vi "Move VI to Subpanel.vi"(8 "error in":errorcluster, 9 "VI name":string, 10 "subpanel tag":string, 11 "state in":T1) -> (0 "error out":errorcluster, 3 "state out":T1)   [LabVIEW 2010, in "NI_SE_Config Front Panel Layout.lvlib"]
uses:
  NI_SE_Config Front Panel Layout.lvlib
  State.ctl
  VI Info.ctl
  VI Panel Layout/VI Panel Layout.lvclass
  VI Panel Layout/Subpanel VI Pair.ctl
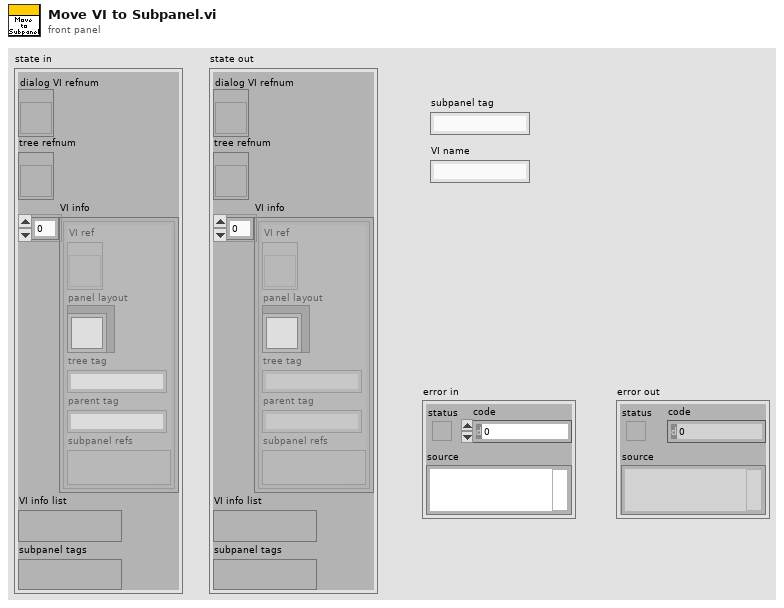
[diagram p1: front panel]
types:
  T1 = typedef "NI_SE_Config Front Panel Layout.lvlib/State.ctl" = cluster{"dialog VI refnum":refnum<vi>, "tree refnum":refnum<vi>, "VI info":T2[], "VI info list":variant, "subpanel tags":variant}
  T2 = typedef "NI_SE_Config Front Panel Layout.lvlib/VI Info.ctl" = cluster{"VI ref":refnum<vi>, "panel layout":refnum<class "VI Panel Layout.lvclass">, "tree tag":string, "parent tag":string, "subpanel refs":variant}
  T3 = typedef "NI_SE_Front Panel Layout.lvlib/VI Panel Layout.lvclass/Subpanel VI Pair.ctl" = cluster{"subpanel UID":i32, "VI name":string, "VI path (rel)":path}
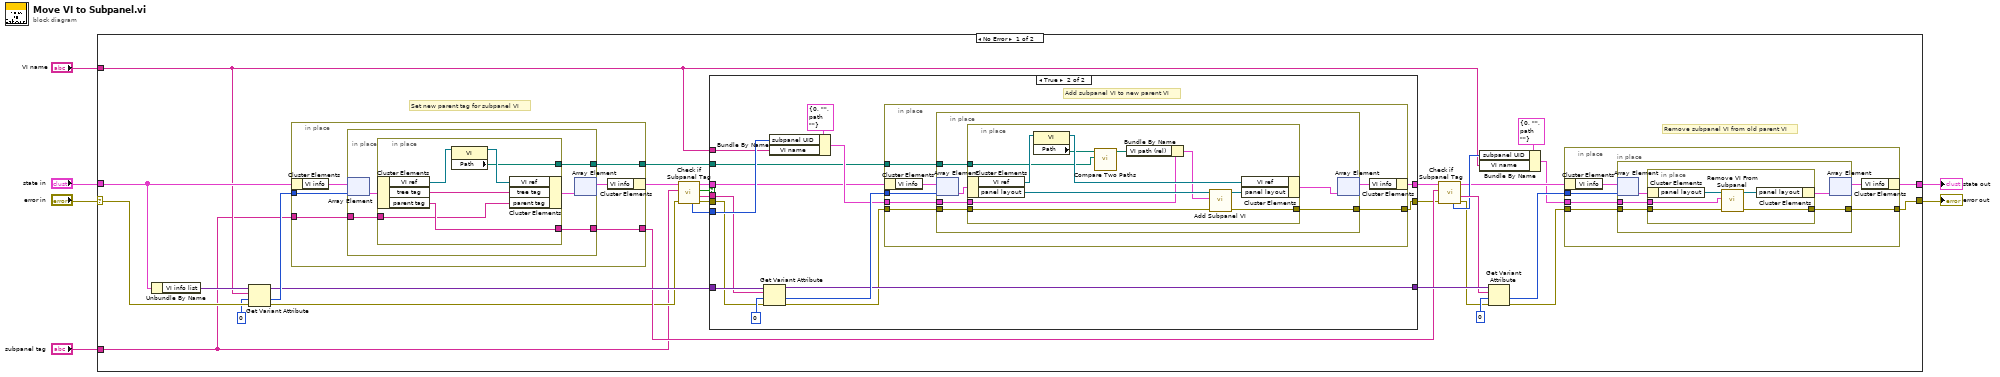
[diagram p0: block diagram]
diagram:
  n1 = case shown="No Error" "error in" {
    selector: "error in" -> [w36 w114]
    tunnel: [w11 w114] -> w5
    tunnel: "subpanel tag" -> [w8 _]
    tunnel: "state in" -> [w37 w113]
    tunnel: "VI name" -> [w20 _]
    tunnel: [w10 w113] -> w1
    frame No Error {
      # "Remove subpanel VI from old parent VI"
      # "Set new parent tag for subpanel VI"
      n2 = Unbundle By Name(w37) -> ("VI info list"=w35:variant)
      n3 = Get Variant Attribute(Variant=w35, name=w20, default value (empty Variant)=0, error in=w36) -> (duplicate Variant=w32:variant, value=w33:i32, error out=w19:errorcluster)  [unwired: 1 out]
      n4 = in-place {
        in-place-border: w33 -> [w99]
        in-place-border: w8 -> [w98]
        in-place-border: [w97] -> w23
        in-place-border: [w96] -> w9
        n5 = in-place-cluster #1(w37) -> ("VI info"=w101:T2[])
        n6 = in-place {
          in-place-border: w98 -> [w104]
          in-place-border: [w103] -> w97
          in-place-border: [w102] -> w96
          n7 = in-place-array #2(w101, w99) -> (w106:T2)
          n8 = in-place {
            in-place-border: w104 -> [w110]
            in-place-border: [w111] -> w103
            in-place-border: [w107] -> w102
            n9 = in-place-cluster #3(w106) -> ("VI ref"=w109:refnum<vi>, "tree tag"=w112:string, "parent tag"=w111:string)
            n10 = property class="VI"(reference=w109) -> (reference out=w108:refnum<vi>, "Path"=w107:path)  [unwired: 1 in, 1 out]
            n11 = in-place-cluster #3("VI ref"=w108, "tree tag"=w112, "parent tag"=w110) -> (w105:T2)
          }
          n12 = in-place-array #2(w105) -> (w100:T2[])  [unwired: 1 out]
        }
        n13 = in-place-cluster #1("VI info"=w100) -> (w31:T1)
      }
      n14 = call "Check if Subpanel Tag.vi"("error in"=w19, "subpanel tag"=w8, "state in"=w31) -> ("error out"=w18:errorcluster, "owning VI name"=w26:string, "found?"=w7:bool, "state out"=w25:T1, "subpanel UID"=w27:i32)  [unwired: 4 in]
      n15 = case shown="True" w7 {
        tunnel: w32 -> [w38 w54]
        tunnel: [w38 w52] -> w30
        tunnel: w27 -> [_ w50]
        tunnel: w26 -> [_ w49]
        tunnel: w25 -> [w40 w47]
        tunnel: [w40 w46] -> w24
        tunnel: w20 -> [_ w45]
        tunnel: w18 -> [w39 w44]
        tunnel: [w39 w43] -> w17
        tunnel: w9 -> [_ w41]
        frame False {
        }
        frame True {
          # "Add subpanel VI to new parent VI"
          n16 = Get Variant Attribute(Variant=w54, name=w49, default value (empty Variant)=0, error in=w44) -> (duplicate Variant=w52:variant, value=w53:i32, error out=w42:errorcluster)  [unwired: 1 out]
          n17 = Bundle By Name(cluster=T3 {"subpanel UID"=0, "VI name"="", "VI path (rel)"=path ""} ("subpanel VI"), "subpanel UID"=w50, "VI name"=w45) -> (w48:T3)
          n18 = in-place {
            in-place-border: w53 -> [w60]
            in-place-border: w48 -> [w59]
            in-place-border: w42 -> [w58]
            in-place-border: [w57] -> w43
            in-place-border: w41 -> [w56]
            n19 = in-place-cluster #4(w47) -> ("VI info"=w62:T2[])
            n20 = in-place {
              in-place-border: w59 -> [w66]
              in-place-border: w58 -> [w65]
              in-place-border: [w64] -> w57
              in-place-border: w56 -> [w63]
              n21 = in-place-array #5(w62, w60) -> (w68:T2)
              n22 = in-place {
                in-place-border: w66 -> [w70]
                in-place-border: w65 -> [w77]
                in-place-border: [w76] -> w64
                in-place-border: w63 -> [w72]
                n23 = in-place-cluster #6(w68) -> ("VI ref"=w75:refnum<vi>, "panel layout"=w79:refnum<class "VI Panel Layout.lvclass">)
                n24 = property class="VI"(reference=w75) -> (reference out=w74:refnum<vi>, "Path"=w73:path)  [unwired: 1 in, 1 out]
                n25 = call <vilib>:"Compare Two Paths.vi"("Path 2"=w72, "Path 1"=w73) -> ("Relative Path from 1 to 2"=w71:path)  [unwired: 6 in, 3 out]
                n26 = Bundle By Name(cluster=w70, "VI path (rel)"=w71) -> (w69:T3)
                n27 = call "Add Subpanel VI.vi"("error in (no error)"=w77, "subpanel VI"=w69, "VI Panel Layout in"=w79) -> ("error out"=w76:errorcluster, "VI Panel Layout out"=w78:refnum<class "VI Panel Layout.lvclass">)  [unwired: 7 in]
                n28 = in-place-cluster #6("VI ref"=w74, "panel layout"=w78) -> (w67:T2)
              }
              n29 = in-place-array #5(w67) -> (w61:T2[])  [unwired: 1 out]
            }
            n30 = in-place-cluster #4("VI info"=w61) -> (w46:T1)
          }
        }
      }
      n31 = call "Check if Subpanel Tag.vi"("error in"=w17, "subpanel tag"=w23, "state in"=w24) -> ("error out"=w16:errorcluster, "owning VI name"=w28:string, "state out"=w15:T1, "subpanel UID"=w21:i32)  [unwired: 4 in, 1 out]
      n32 = Bundle By Name(cluster=T3 {"subpanel UID"=0, "VI name"="", "VI path (rel)"=path ""} ("subpanel VI"), "subpanel UID"=w21, "VI name"=w20) -> (w12:T3)
      n33 = Get Variant Attribute(Variant=w30, name=w28, default value (empty Variant)=0, error in=w16) -> (value=w13:i32, error out=w14:errorcluster)  [unwired: 2 out]
      n34 = in-place {
        in-place-border: w13 -> [w83]
        in-place-border: w12 -> [w82]
        in-place-border: w14 -> [w81]
        in-place-border: [w80] -> w11
        n35 = in-place-cluster #7(w15) -> ("VI info"=w85:T2[])
        n36 = in-place {
          in-place-border: w82 -> [w88]
          in-place-border: w81 -> [w87]
          in-place-border: [w86] -> w80
          n37 = in-place-array #8(w85, w83) -> (w90:T2)
          n38 = in-place {
            in-place-border: w88 -> [w92]
            in-place-border: w87 -> [w93]
            in-place-border: [w91] -> w86
            n39 = in-place-cluster #9(w90) -> ("panel layout"=w95:refnum<class "VI Panel Layout.lvclass">)
            n40 = call "Remove VI From Subpanel.vi"("error in (no error)"=w93, "subpanel VI"=w92, "VI Panel Layout in"=w95) -> ("error out"=w91:errorcluster, "VI Panel Layout out"=w94:refnum<class "VI Panel Layout.lvclass">)  [unwired: 7 in]
            n41 = in-place-cluster #9("panel layout"=w94) -> (w89:T2)
          }
          n42 = in-place-array #8(w89) -> (w84:T2[])  [unwired: 1 out]
        }
        n43 = in-place-cluster #7("VI info"=w84) -> (w10:T1)
      }
    }
    frame Error {
    }
  }
  "state out" <- w1
  "error out" <- w5
